vi "Find Answer.vi"(10 "P1":bool, 11 "Circular Buffer in":refnum<class "Circular Buffer.lvclass">) -> (2 "Answer":i64, 3 "Circular Buffer out":refnum<class "Circular Buffer.lvclass">)   [LabVIEW 2023, in "d20.lvlib" / "Circular Buffer.lvclass"]
uses:
  Circular Buffer.lvclass
  Circular Buffer.lvclass/Circular Buffer.ctl
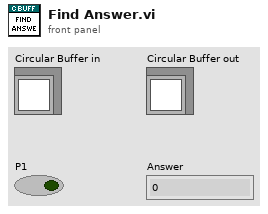
[diagram p1: front panel]
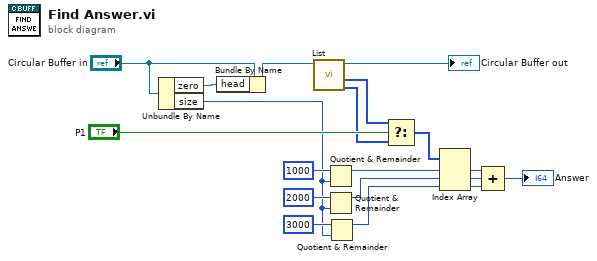
[diagram p0: block diagram]
diagram:
  n1 = Unbundle By Name("Circular Buffer in") -> ("zero"=w2:refnum<data-value>, "size"=w4:i64)
  n2 = Bundle By Name(cluster="Circular Buffer in", "head"=w2) -> (w3:refnum<class "Circular Buffer.lvclass">)
  n3 = call "List.vi"("Circular Buffer in"=w3) -> ("Decryption List"=w1:i64[], "Shift List"=w6:i64[], "Circular Buffer out"=→"Circular Buffer out":refnum<class "Circular Buffer.lvclass">)  [unwired: 7 in, 1 out]
  n4 = Quotient & Remainder(x=i64 1000, y=w4) -> (x-y*floor(x/y)=w10:i64)  [unwired: 1 out]
  n5 = Quotient & Remainder(x=i64 2000, y=w4) -> (x-y*floor(x/y)=w12:i64)  [unwired: 1 out]
  n6 = Quotient & Remainder(x=i64 3000, y=w4) -> (x-y*floor(x/y)=w14:i64)  [unwired: 1 out]
  n7 = Select(t=w6, s="P1", f=w1) -> (s? t:f=w7:i64[])
  n8 = Index Array(array=w7, index #1=w10, index #2=w12, index #3=w14) -> (element #1=w15:i64, element #2=w16:i64, element #3=w17:i64)
  n9 = Compound Arithmetic op=ADD(w15, w16, w17) -> (→"Answer":i64)
